vi "main.vi"() -> ()   [LabVIEW 2015]
uses:
  <vilib>/Bitlis-MEN/Parallel Stop/Software/Stop_Command.ctl
  <vilib>/DAQmx/read.llb/DAQmx Read (Analog 2D DBL NChan NSamp).vi
  <vilib>/Analysis/baseanly.llb/Mean (DBL).vi
  <vilib>/DAQmx/miscellaneous.llb/DAQmx Fill In Error Info.vi
  <vilib>/Utility/file.llb/Write Delimited Spreadsheet (DBL).vi
  <vilib>/Utility/file.llb/Write Delimited Spreadsheet (string).vi
  <vilib>/Analysis/NI_AALBase.lvlib
panel:
  in  "Tab Control":enum32{"Main", "Page 2"}(tab)
  in  "Enabled 1":bool=TRUE
  in  "Scale 1":tag="CO2_5000PPM"
  in  "AI Channel 1":tag="KAPDAQ/ai0"
  in  "Label 1":string="CO2"
  in  "Enabled 2":bool
  in  "Scale 2":tag="SO2_500"
  in  "AI Channel 2":tag="KAPDAQ/ai1"
  in  "Label 2":string="SO2"
  in  "Enabled 3":bool
  in  "Scale 3":tag="CO_1PPM"
  in  "AI Channel 3":tag="KAPDAQ/ai2"
  in  "Label 3":string="CO"
  in  "Enabled 4":bool
  in  "Scale 4":tag="Ozone_500"
  in  "AI Channel 4":tag="KAPDAQ/ai3"
  in  "Label 4":string="O3"
  in  "Enabled 5":bool
  in  "Scale 5":tag="NO_200ppb"
  in  "AI Channel 5":tag="KAPDAQ/ai4"
  in  "Label 5":string="NO"
  in  "Enabled 6":bool
  in  "Scale 6":tag="NO2_200ppb"
  in  "AI Channel 6":tag="KAPDAQ/ai5"
  in  "Label 6":string="NO2"
  in  "Enabled 7":bool
  in  "Scale 7":tag="NOx_200ppb"
  in  "AI Channel 7":tag="KAPDAQ/ai6"
  in  "Label 7":string="NOx"
  in  "Enabled 8":bool
  in  "Scale 8":tag
  in  "AI Channel 8":tag="KAPDAQ/ai7"
  in  "Label 8":string
  out "State":enum16{"Sample", "Shutdown", "Initialize"}(ring)=enum."Initialize"
  in  "Stop Button":bool
  in  "Sampling Freq (Hz)":dbl=1.0
  in  "number of samples per channel":i32=-1
  out "Results":dbl[](array[numeric]) format="%_3g"
  out "Labels":string[](array[string])
  out "error out":errorcluster
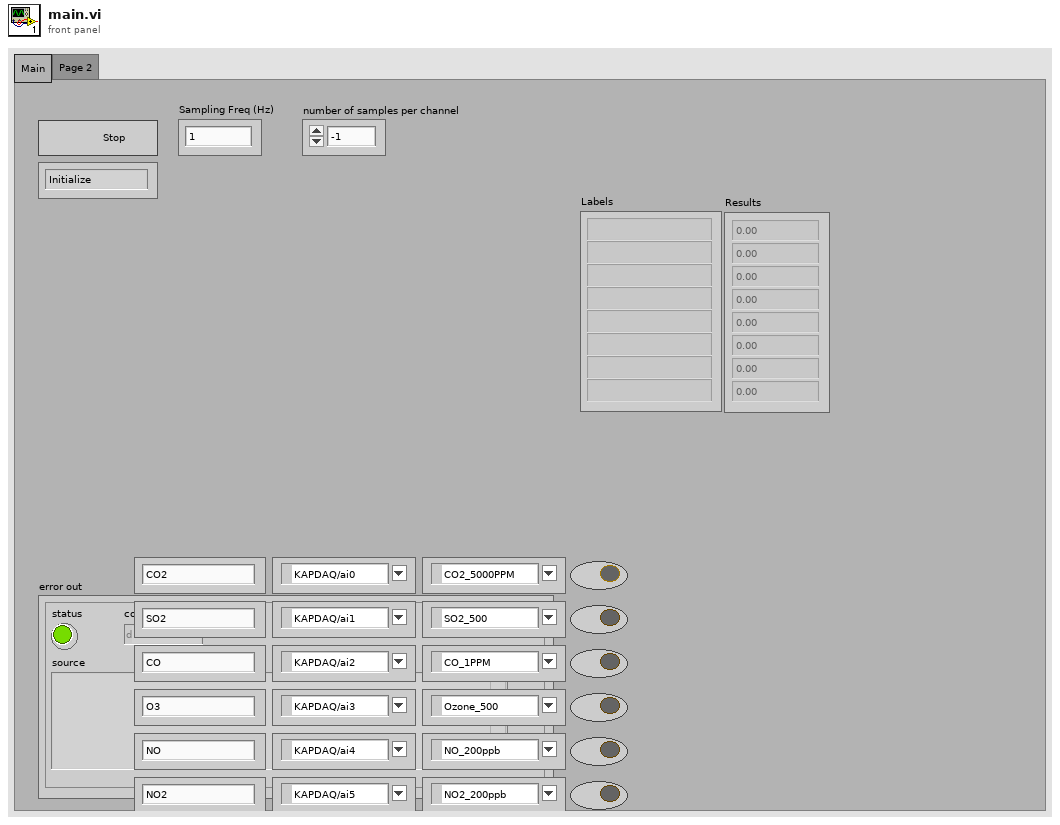
[diagram p1: front panel]
types:
  T1 = cluster{"Label":string, "Channel":tag, "DAQmx Scale Name":tag, "Enabled":bool}[]
  T2 = typedef "Stop_Command.ctl" = enum16{"Reset", "Read", "Write", "Close"}
  T3 = cluster{"Label":string, "Channel":tag, "DAQmx Scale Name":tag, "Enabled":bool}
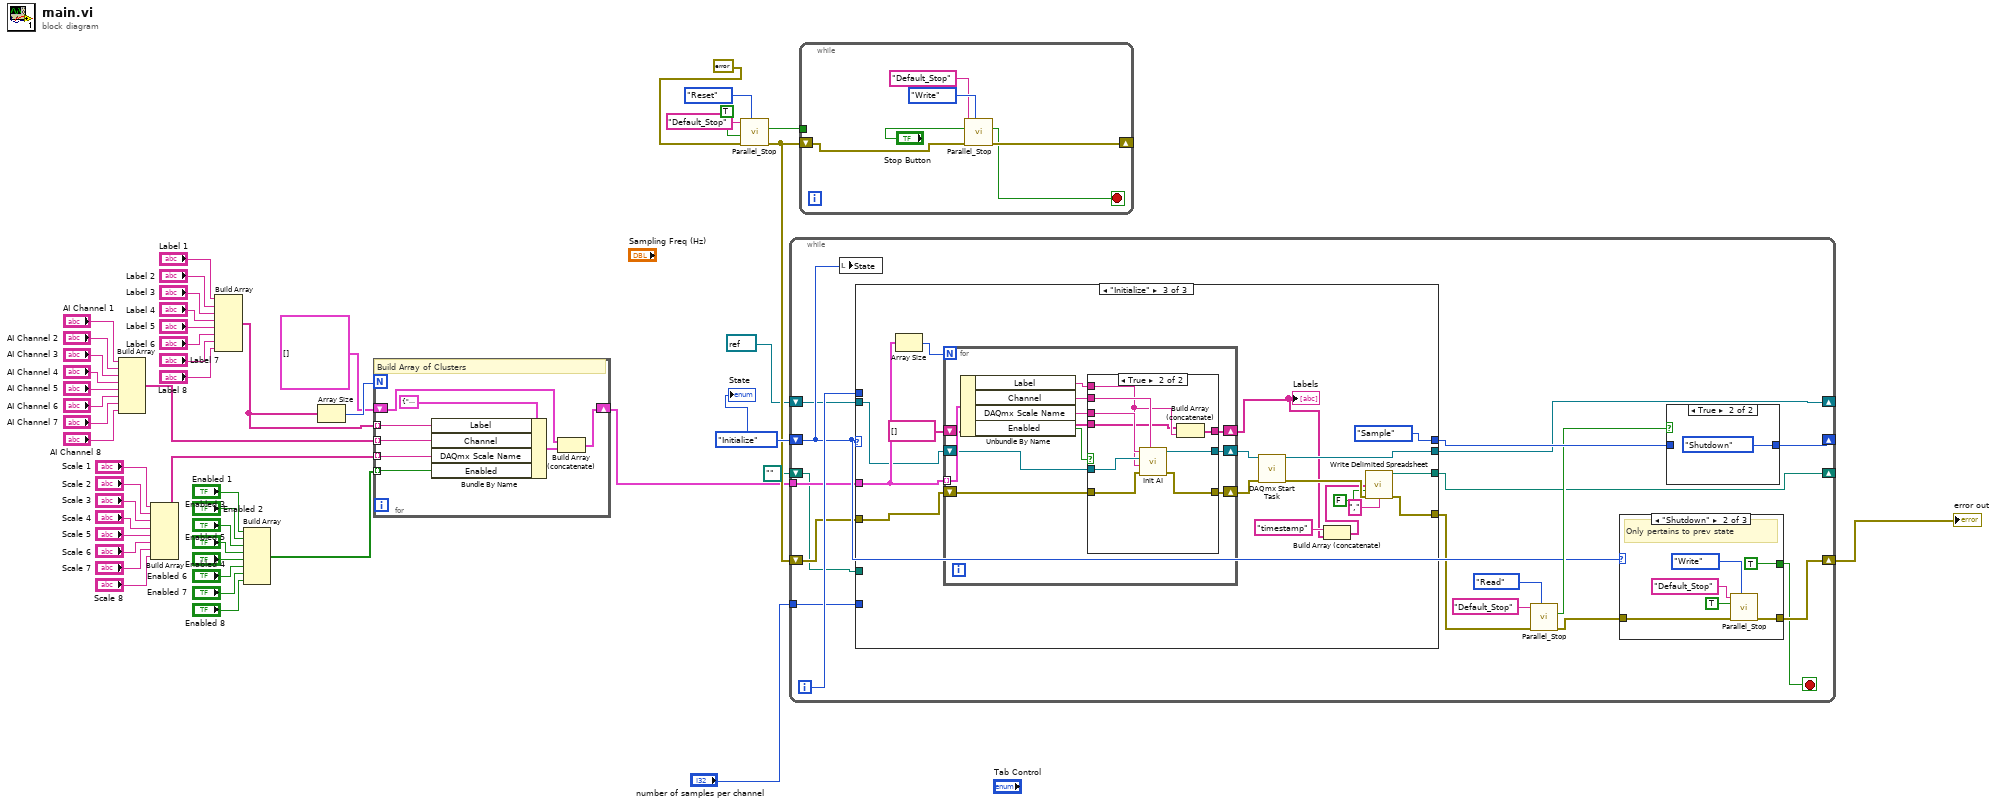
[diagram p0: block diagram]
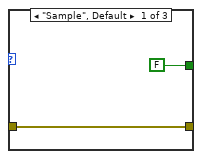
[diagram p3: hidden frame]
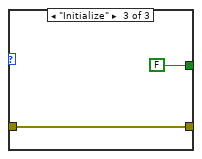
[diagram p4: hidden frame]
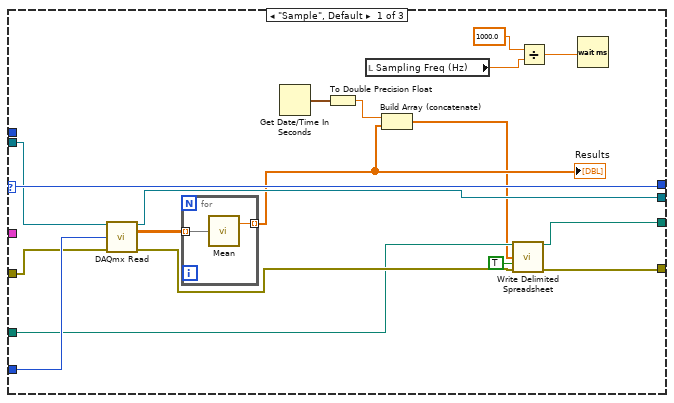
[diagram p5: hidden frame]
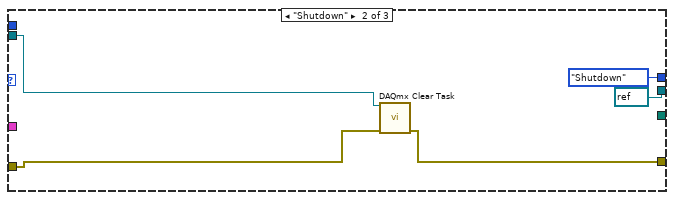
[diagram p6: hidden frame]
diagram:
  w50 = enum16{"Sample", "Shutdown", "Initialize"}."Initialize"
  n1 = Build Array("AI Channel 1", "AI Channel 2", "AI Channel 3", "AI Channel 4", "AI Channel 5", "AI Channel 6", "AI Channel 7", "AI Channel 8") -> (w30:tag[])
  n2 = Build Array("Scale 1", "Scale 2", "Scale 3", "Scale 4", "Scale 5", "Scale 6", "Scale 7", "Scale 8") -> (w29:tag[])
  n3 = Build Array("Label 1", "Label 2", "Label 3", "Label 4", "Label 5", "Label 6", "Label 7", "Label 8") -> (w31:string[])
  n4 = Build Array("Enabled 1", "Enabled 2", "Enabled 3", "Enabled 4", "Enabled 5", "Enabled 6", "Enabled 7", "Enabled 8") -> (w28:bool[])
  n5 = Array Size(array=w31) -> (size(s)=w32:i32)
  n6 = for {
    N: w32 -> [_]
    tunnel: w31 -> [w54] mode=indexing
    tunnel: w30 -> [w53] mode=indexing
    tunnel: w29 -> [w52] mode=indexing
    tunnel: w28 -> [w51] mode=indexing
    shift-right: [w56] -> w26
    shift-left: T1 [] -> [w55]
    # "Build Array of Clusters"
    n7 = Bundle By Name(cluster=T3 {"Label"="", "Channel"="", "DAQmx Scale Name"="", "Enabled"=TRUE}, "Label"=w54, "Channel"=w53, "DAQmx Scale Name"=w52, "Enabled"=w51) -> (w57:T3)
    n8 = Build Array (concatenate)(w55, w57) -> (w56:T1)
  }
  n9 = call <vilib>:"Parallel_Stop.vi"("Command"=Stop_Command."Reset", "error in (no error)"=errorcluster {"status"=FALSE, "code"=0, "source"=""}, "Stop on Error? (T)"=TRUE, "Name"="Default_Stop") -> ("error out"=w44:errorcluster, "Latched Stop"=w46:bool)  [unwired: 6 in]
  n10 = while {
    shift-right: [w69] -> w43
    shift-left: w44 -> [w66]
    shift-right: [w73] -> _
    shift-left: w50 -> [w67]
    shift-right: [w64] -> _
    shift-left: refnum<k21> refnum ("task out") -> [w63]
    tunnel: "number of samples per channel" -> [w62]
    tunnel: w26 -> [w61]
    shift-right: [w60] -> _
    shift-left: path "" ("new file path (Not A Path if cancelled)") -> [w59]
    i -> [w74]
    stop <- w68 stop-if-true
    n11 = local write "State"(w67) -> ()
    n12 = case shown="\"Initialize\"" w67 {
      selector: w67 -> [w106 _ _]
      tunnel: [w106 enum16{"Sample", "Shutdown", "Initialize"}."Shutdown" enum16{"Sample", "Shutdown", "Initialize"}."Sample"] -> w72
      tunnel: w74 -> [_ _ _]
      tunnel: w66 -> [w103 w111 w126]
      tunnel: [w96 w110 w120] -> w65
      tunnel: [w102 refnum<k21> refnum ("task out") w129] -> w64
      tunnel: w63 -> [w105 w112 w125]
      tunnel: w62 -> [w104 _ _]
      tunnel: w61 -> [_ _ w127]
      tunnel: [w95 _ w114] -> w60
      tunnel: w59 -> [w94 _ _]
      frame "Sample", Default {
        n13 = call-poly <vilib>:"DAQmx Read.vi"("task/channels in"=w105, "number of samples per channel"=w104, "error in"=w103) -> ("task out"=w102:refnum<k21>, "data"=w101:dbl[][], "error out"=w97:errorcluster)  [unwired: 10 in]
        n14 = for {
          tunnel: w101 -> [w108] mode=indexing
          tunnel: [w107] -> w92 mode=indexing
          n15 = call-poly <vilib>:"Mean.vi"("X"=w108) -> ("mean"=w107:dbl)  [unwired: 1 out]
        }
        "Results" <- w92
        n16 = Get Date/Time In Seconds() -> (seconds since 1Jan1904=w91:timestamp)
        n17 = To Double Precision Float(number=w91) -> (double precision float=w90:dbl)
        n18 = local read "Sampling Freq (Hz)"() -> (w99:dbl)
        n19 = Build Array (concatenate)(w90, w92) -> (w89:dbl[])
        n20 = call-poly <vilib>:"Write Delimited Spreadsheet.vi"("file path (dialog if empty)"=w94, "1D data"=w89, "append to file? (F)"=TRUE, "error in (no error)"=w97) -> ("new file path (Not A Path if cancelled)"=w95:path, "error out"=w96:errorcluster)  [unwired: 10 in]
        n21 = Divide(x=1000.0, y=w99) -> (x/y=w100:dbl)
        n22 = Wait (ms)(milliseconds to wait=w100) -> ()  [unwired: 1 out]
      }
      frame "Shutdown" {
        n23 = call <vilib>:"DAQmx Clear Task.vi"("task in"=w112, "error in"=w111) -> ("error out"=w110:errorcluster)  [unwired: 13 in]
      }
      frame "Initialize" {
        n24 = Array Size(array=w127) -> (size(s)=w128:i32)
        n25 = for {
          N: w128 -> [_]
          tunnel: w127 -> [w141] mode=indexing
          shift-right: [w136] -> w124
          shift-left: w126 -> [w137]
          shift-right: [w134] -> w123
          shift-left: w125 -> [w133]
          shift-right: [w132] -> w116
          shift-left: string[] [] -> [w131]
          n26 = Unbundle By Name(w141) -> ("Label"=w139:string, "Channel"=w135:tag, "DAQmx Scale Name"=w138:tag, "Enabled"=w140:bool)
          n27 = case shown="True" w140 {
            tunnel: w139 -> [_ w147]
            tunnel: w138 -> [_ w153]
            tunnel: w137 -> [w143 w152]
            tunnel: [w143 w151] -> w136
            tunnel: w135 -> [_ w150]
            tunnel: [w144 w149] -> w134
            tunnel: w133 -> [w144 w148]
            tunnel: [w142 w146] -> w132
            tunnel: w131 -> [w142 w145]
            frame False {
            }
            frame True {
              n28 = call "Init AI.vi"("DAQmx Physical Channel"=w150, "error in (no error)"=w152, "label"=w147, "task in"=w148, "DAQmx Scale Name"=w153) -> ("error out"=w151:errorcluster, "Task Out"=w149:refnum<k21>)  [unwired: 5 in]
              n29 = Build Array (concatenate)(w145, w147) -> (w146:string[])
            }
          }
        }
        "Labels" <- w116
        n30 = call <vilib>:"DAQmx Start Task.vi"("task/channels in"=w123, "error in"=w124) -> ("task out"=w129:refnum<k21>, "error out"=w121:errorcluster)  [unwired: 12 in]
        n31 = Build Array (concatenate)("timestamp" ("string"), w116) -> (w115:string[])
        n32 = call-poly <vilib>:"Write Delimited Spreadsheet.vi"("1D data"=w115, "append to file? (F)"=FALSE, "error in (no error)"=w121, "delimiter (\\t)"="," ("delimiter (\\t)")) -> ("new file path (Not A Path if cancelled)"=w114:path, "error out"=w120:errorcluster)  [unwired: 10 in]
      }
    }
    n33 = call <vilib>:"Parallel_Stop.vi"("Command"=Stop_Command."Read", "error in (no error)"=w65, "Name"="Default_Stop") -> ("error out"=w70:errorcluster, "Latched Stop"=w71:bool)  [unwired: 7 in]
    n34 = case shown="\"Shutdown\"" w67 {
      tunnel: w70 -> [w80 w83 w88]
      tunnel: [w80 w82 w88] -> w69
      tunnel: [FALSE TRUE FALSE] -> w68
      frame "Sample", Default {
      }
      frame "Shutdown" {
        # "Only pertains to prev state"
        n35 = call <vilib>:"Parallel_Stop.vi"("Command"=Stop_Command."Write", "error in (no error)"=w83, "Stop?"=TRUE, "Name"="Default_Stop") -> ("error out"=w82:errorcluster)  [unwired: 6 in, 1 out]
      }
      frame "Initialize" {
      }
    }
    n36 = case shown="True" w71 {
      tunnel: [w77 enum16{"Sample", "Shutdown", "Initialize"}."Shutdown"] -> w73
      tunnel: w72 -> [w77 _]
      frame False {
      }
      frame True {
      }
    }
  }
  "error out" <- w43
  n37 = while {
    tunnel: w46 -> [_]
    shift-right: [w158] -> _
    shift-left: w44 -> [w157]
    stop <- w156 stop-if-true
    n38 = call <vilib>:"Parallel_Stop.vi"("Command"=Stop_Command."Write", "error in (no error)"=w157, "Stop?"="Stop Button", "Name"="Default_Stop") -> ("error out"=w158:errorcluster, "Latched Stop"=w156:bool)  [unwired: 6 in]
  }
  "State" <- w50
